vi "Save Batt Data.vi"(6 "Error In":errorcluster, 8 "Shim #":i32, 9 "Battery Capture":u64) -> (0 "error out":errorcluster, 2 "Pass/Fail #":i32, 3 "Pass?":bool)   [LabVIEW 2015]
uses:
  <vilib>/Utility/NIReport.llb/NI_report.lvclass
  <vilib>/Utility/NIReport.llb/Excel/NI_Excel.lvclass
  <vilib>/addons/_office/NI_ReportGenerationToolkit.lvlib
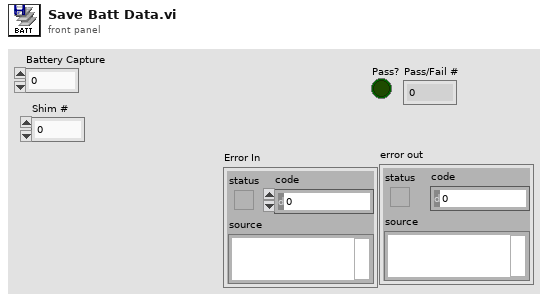
[diagram p1: front panel]
types:
  T1 = enum16{"maximized", "minimized", "normal", "no change"}
  T2 = enum16{"Standard Report", "HTML", "Word", "Excel"}
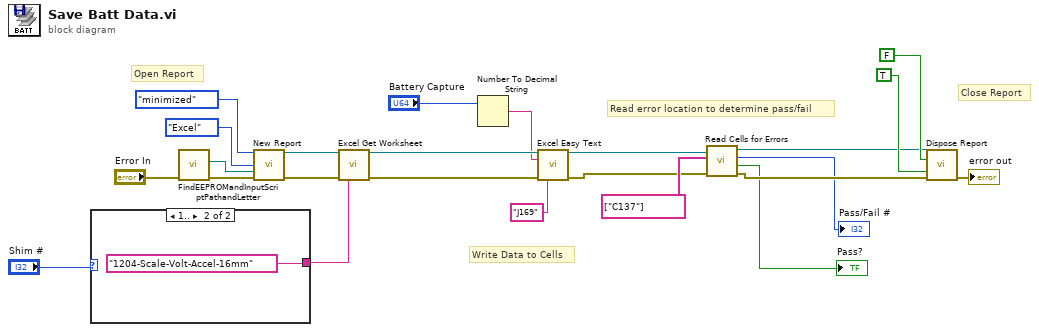
[diagram p0: block diagram]
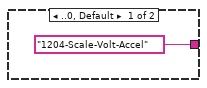
[diagram p2: hidden frame]
diagram:
  # "Open Report"
  # "Close Report"
  # "Read error location to determine pass/fail"
  # "Write Data to Cells"
  n1 = case shown="1.." "Shim #" {
    tunnel: ["1204-Scale-Volt-Accel" ("name (\"\")") "1204-Scale-Volt-Accel-16mm" ("name (\"\")")] -> w2
    frame ..0, Default {
    }
    frame 1.. {
    }
  }
  n2 = call "FindEEPROMandInputScriptPathandLetter.vi"("Error In"="Error In") -> ("Error Out"=w16:errorcluster, "Engr Result Path"=w20:path)  [unwired: 6 in, 1 out]
  n3 = call <vilib>:"New Report.vi"("window state (normal)"=T1."minimized", "report type"=T2."Excel", "template (empty)"=w20, "error in (no error)"=w16) -> ("report out"=w18:refnum<class "NI_report.lvclass">, "error out"=w19:errorcluster)  [unwired: 10 in]
  n4 = call <vilib>:"Excel Get Worksheet.vi"("report in"=w18, "error in (no error)"=w19, "name (\"\")"=w2) -> ("report out"=w14:refnum<class "NI_report.lvclass">, "error out"=w13:errorcluster)  [unwired: 11 in]
  n5 = Number To Decimal String(number="Battery Capture") -> (decimal integer string=w3:string)  [unwired: 1 in]
  n6 = call <vilib>:"Excel Easy Text.vi"("report in"=w14, "text"=w3, "error in (no error)"=w13, "name (\"\")"="J169") -> ("report out"=w12:refnum<class "NI_report.lvclass">, "error out"=w10:errorcluster)  [unwired: 7 in, 3 out]
  n7 = call "Read Cells for Errors.vi"("error in (no error)"=w10, "Error Cells (ex:A12)"=string[] ["C137"] ("Array"), "NI_report in"=w12) -> ("error out"=w8:errorcluster, "Pass?"=→"Pass?":bool, "Error Code"=→"Pass/Fail #":i32, "NI_report out"=w9:refnum<class "NI_report.lvclass">)  [unwired: 5 in]
  n8 = call-dynamic "Dispose Report.vi"("report in"=w9, "wait until printing completed? (T)"=FALSE, "save changes? (F)"=TRUE, "error in (no error)"=w8) -> ("error out"=→"error out":errorcluster)  [unwired: 11 in]
